vi "adam-analog-input.vi"(0 "VISA Refnum in":refnum<visa-resource-name>, 1 "Chassis Settings":T1, 9 "chassis-slot":i32, 11 "error in (no error)":errorcluster, 12 "last cmd in":string, 13 "last read buffer":string) -> (4 "VISA Refnum out":refnum<visa-resource-name>, 6 "Analog Inputs":T2, 8 "cmd out":string, 10 "read-buffer out":string, 14 "cmd aknowledged":bool, 15 "error out":errorcluster)   [LabVIEW 2020]
uses:
  controls/analog-input-cluster.ctl
  controls/adam-5000-serial-settings.ctl
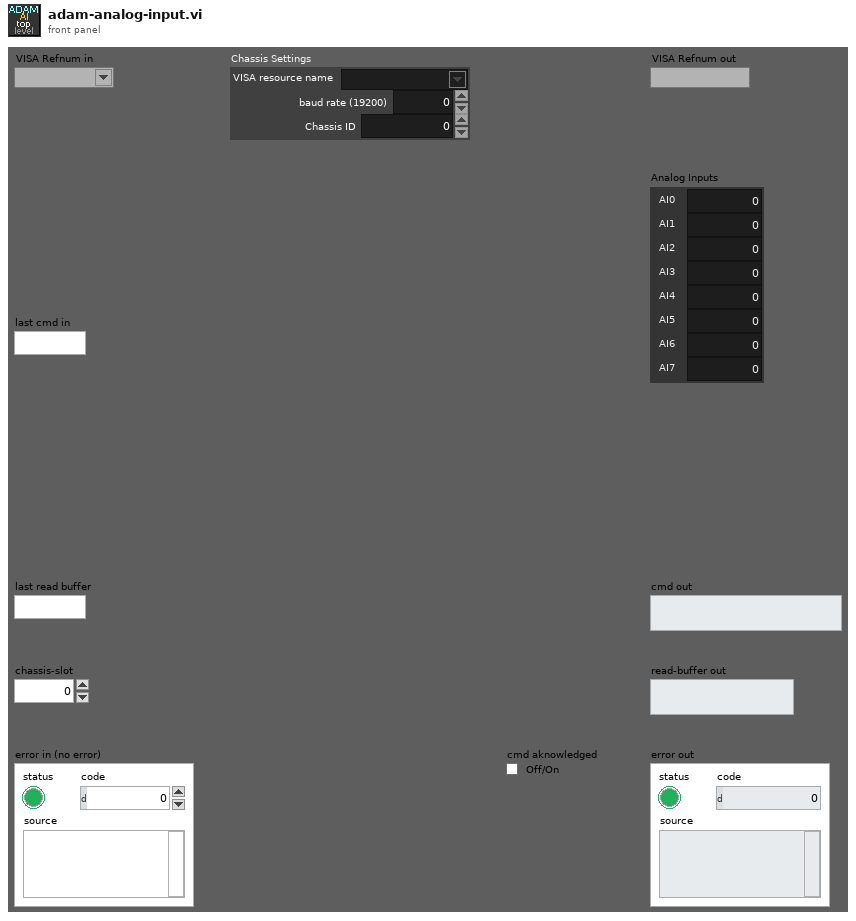
[diagram p1: front panel]
types:
  T1 = typedef "adam-5000-serial-settings.ctl" = cluster{"VISA resource name":refnum<visa-resource-name>, "baud rate (19200)":u32, "Chassis ID":u8}
  T2 = typedef "analog-input-cluster.ctl" = cluster{"AI0":dbl, "AI1":dbl, "AI2":dbl, "AI3":dbl, "AI4":dbl, "AI5":dbl, "AI6":dbl, "AI7":dbl}
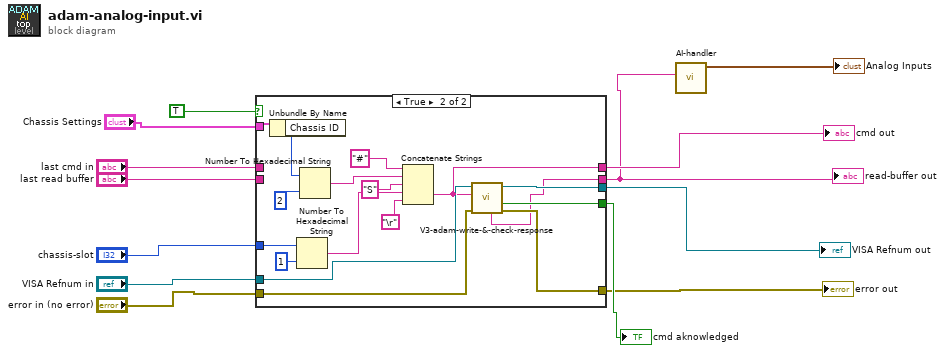
[diagram p0: block diagram]
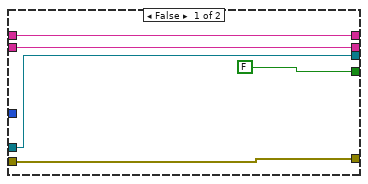
[diagram p2: hidden frame]
diagram:
  n1 = case shown="True" TRUE {
    tunnel: "VISA Refnum in" -> [w18 w31]
    tunnel: "error in (no error)" -> [w16 w30]
    tunnel: [w16 w29] -> w4
    tunnel: [w18 w28] -> w5
    tunnel: [FALSE ("cmd aknowledged") w27] -> w13
    tunnel: [w15 w19] -> w10
    tunnel: [w14 w26] -> w12
    tunnel: "Chassis Settings" -> [_ w24]
    tunnel: "chassis-slot" -> [_ w23]
    tunnel: "last read buffer" -> [w15 _]
    tunnel: "last cmd in" -> [w14 _]
    frame False {
    }
    frame True {
      n2 = Unbundle By Name(w24) -> ("Chassis ID"=w35:u8)
      n3 = Number To Hexadecimal String(1:i16 1 ("width (-)"), 2:w23) -> (0:w21:string)
      n4 = Number To Hexadecimal String(1:i16 2 ("width (-)"), 2:w35) -> (0:w33:string)
      n5 = Concatenate Strings("#" ("string"), w33, "S" ("string"), w21, "\r") -> (w26:string)
      n6 = call "V3-adam-write-&-check-response.vi"("error in (no error)"=w30, "write buffer"=w26, "VISA resource name"=w31) -> ("error out"=w29:errorcluster, "cmd aknowledged"=w27:bool, "VISA resource name out"=w28:refnum<visa-resource-name>, "read buffer"=w19:string)  [unwired: 4 in, 1 out]
    }
  }
  "cmd aknowledged" <- w13
  "cmd out" <- w12
  "read-buffer out" <- w10
  "VISA Refnum out" <- w5
  "error out" <- w4
  n7 = call "AI-handler.vi"("read buffer in"=w10) -> ("Analog Inputs"=→"Analog Inputs":T2)  [unwired: 10 in]
